vi "Read BombedWallParams.vi"(8 "error in (no error)":errorcluster, 11 "RoomWithBomb":refnum<class "RoomWithBomb.lvclass">) -> (0 "error out":errorcluster, 2 "RoomWithBombParams":T1, 3 "RoomWithBomb":refnum<class "RoomWithBomb.lvclass">)   [LabVIEW 2020, in "RoomWithBomb.lvclass"]
uses:
  RoomWithBomb.lvclass
  TypeDef/RoomWithBombParams.ctl
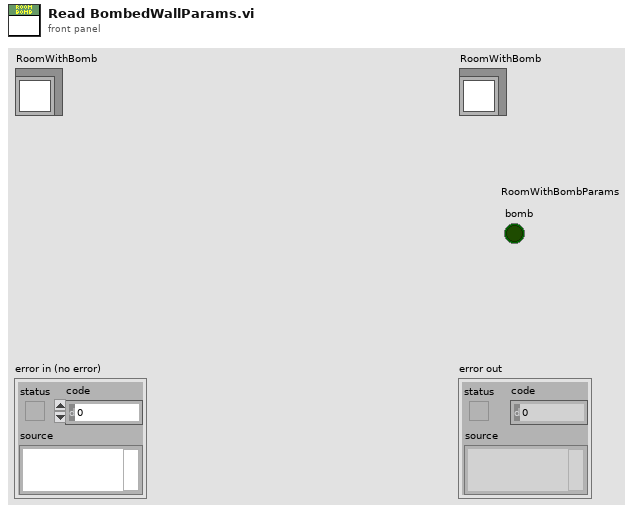
[diagram p1: front panel]
types:
  T1 = typedef "RoomWithBomb.lvclass/RoomWithBombParams.ctl" = cluster{"bomb":bool}
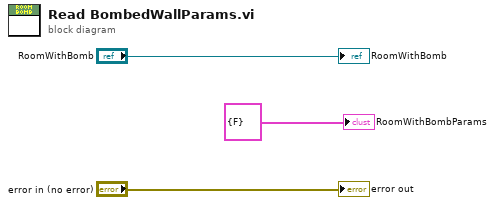
[diagram p0: block diagram]
diagram:
  "error out" <- "error in (no error)"
  "RoomWithBomb" <- "RoomWithBomb"
  "RoomWithBombParams" <- T1 {"bomb"=FALSE} ("<ClassName>Params")
